vi "Save Recall Sequence.vi"(6 "Sequence Operation (0: Recall)":i32(ring) items=["Recall", "Save"], 7 "File Location (0: Internal)":i32(ring) items=["Internal", "External"], 8 "error in (no error)":errorcluster {"code" format="%.0x"}, 9 "Sequence File Path (sequence1.seq)":string="sequence1.seq", 10 "Channel Name (1)":string="1", 11 "VISA resource name":refnum<visa-resource-name>) -> (0 "error out":errorcluster {"code" format="%.0x"}, 3 "VISA resource name out":refnum<visa-resource-name>)   [LabVIEW 2014, in "Agilent N6700 Series.lvlib"]
doc: "Recalls or saves the sequence settings on the N6705B model.\n\n<b>Note:</b>\nThis VI only applies to the N6705B and N6705C DC Power Analyzer."
uses:
  Agilent N6700 Series.lvlib
panel:
  # "The sequence file path must include a .seq file extension \nand can only be saved to an existing folder."
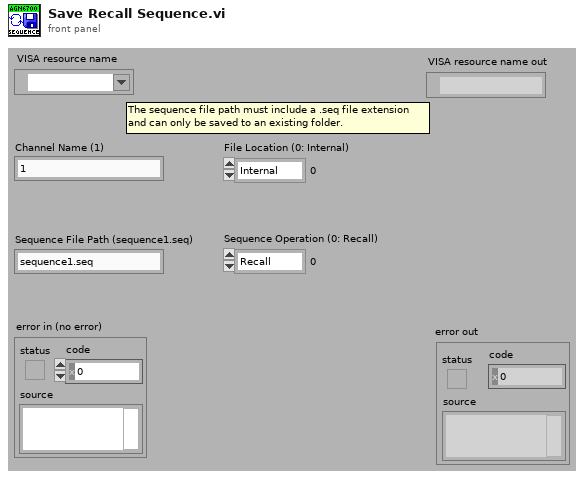
[diagram p1: front panel]
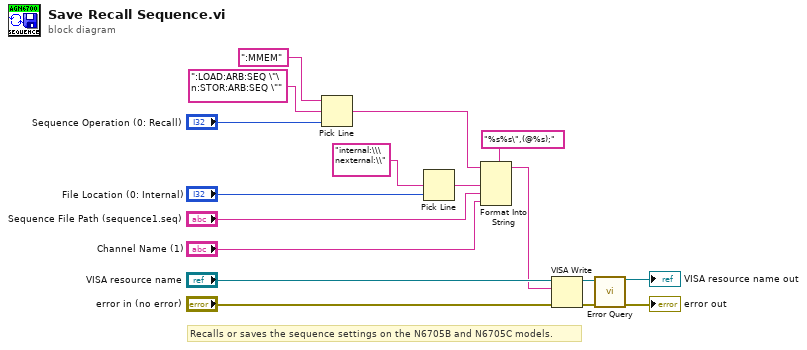
[diagram p0: block diagram]
diagram:
  # "Recalls or saves the sequence settings on the N6705B and N6705C models."
  n1 = Pick Line(string ("")=":MMEM", multi-line string=":LOAD:ARB:SEQ \"\n:STOR:ARB:SEQ \"", line index="Sequence Operation (0: Recall)") -> (output string=w7:string)
  n2 = Pick Line(multi-line string="internal:\\\nexternal:\\", line index="File Location (0: Internal)") -> (output string=w2:string)  [unwired: 1 in]
  n3 = Format Into String(format string="%s%s\",(@%s);", initial string=w7, w2, "Sequence File Path (sequence1.seq)", "Channel Name (1)") -> (resulting string=w6:string)  [unwired: 1 in, 1 out]
  n4 = VISA Write(VISA resource name="VISA resource name", write buffer=w6, error in (no error)="error in (no error)") -> (VISA resource name out=w13:refnum<visa-resource-name>, error out=w12:errorcluster)  [unwired: 1 out]
  n5 = call "Error Query.vi"("VISA resource name"=w13, "error in (no error)"=w12) -> ("VISA resource name out"=→"VISA resource name out":refnum<visa-resource-name>, "error out"=→"error out":errorcluster)  [unwired: 10 in, 2 out]
